vi "CalDiaVelAll.vi"() -> ()   [LabVIEW 2017]
uses:
  <vilib>/Utility/file.llb/Write Delimited Spreadsheet (string).vi
  <vilib>/Utility/file.llb/Write Delimited Spreadsheet (DBL).vi
panel:
  in  "Velocity Results File":path
  in  "Diameter Results File":path
  in  "Calibration (1 pixel = ?um)":dbl=1.45
  out "Measurment Progress":u8(slide) scale=0.0..36.0
  out "Quantifying":dbl
  out "Total Video Segments to Quantify":dbl
  # "This VI performs diameter and velocity measurements of all videos in the selected folder. The user is prompted to select the folder after which they choose a point on the top vessel wall for all the segments then a point on the bottom vessel wall. The VI then runs through all the segments and outputs the values into two text files 'Diameter' and 'Velocity'. Due to dependencies this VI is currently set to use frame 5000 as a template"
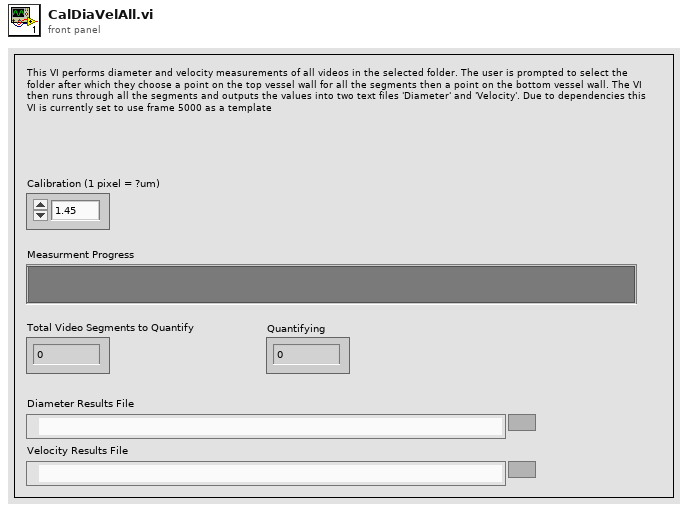
[diagram p1: front panel]
types:
  T1 = typedef "IMAQ AVI2 Refnum.ctl" = refnum<k20>
  T2 = typedef "IMAQ Image.ctl" = refnum<image>
  T3 = typedef "IMAQ Point" = cluster{"X":sgl, "Y":sgl}
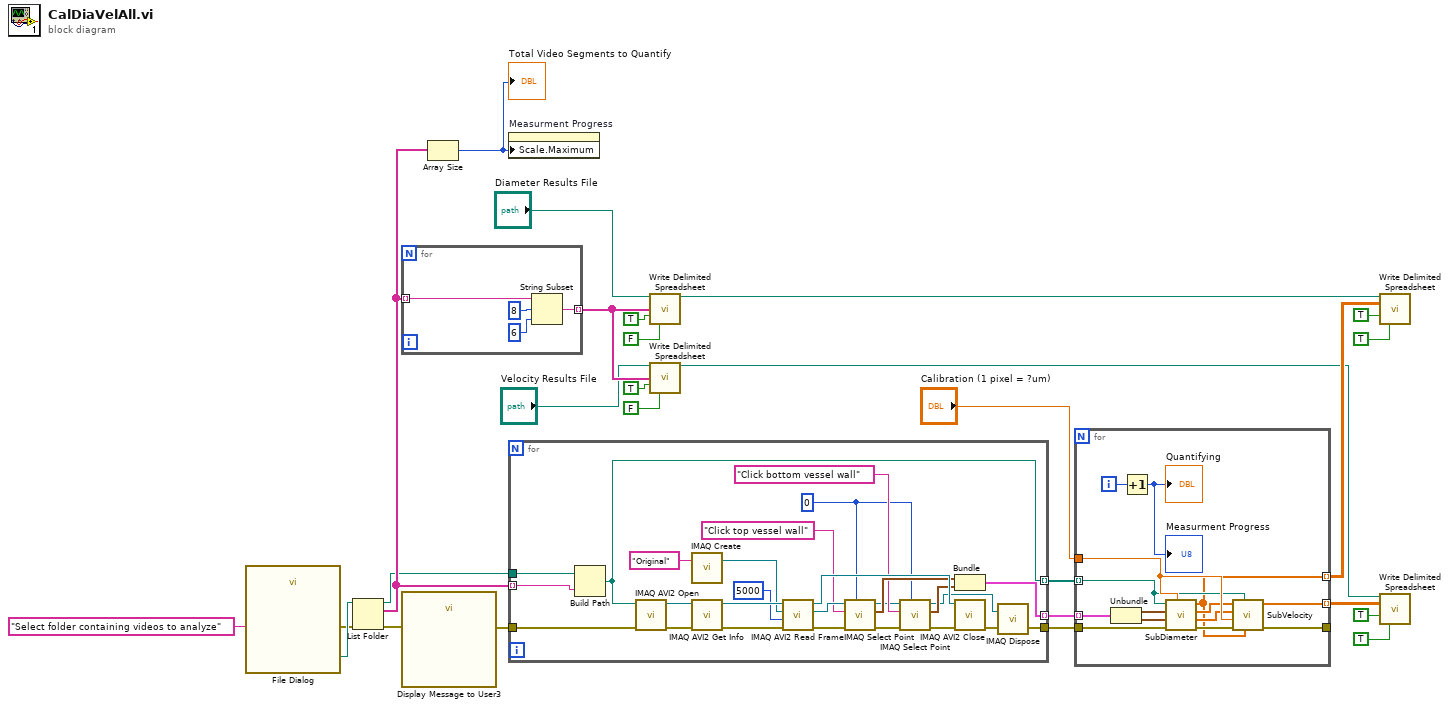
[diagram p0: block diagram]
diagram:
  n1 = call "File Dialog"("prompt"="Select folder containing videos to analyze") -> ("selected path"=w26:path, "error out"=w25:errorcluster)  [unwired: 11 in, 2 out]
  n2 = List Folder(path=w26, error in=w25) -> (path out=w9:path, filenames=w10:string[], error out=w12:errorcluster)  [unwired: 2 in, 1 out]
  n3 = for {
    tunnel: w10 -> [w31] mode=indexing
    tunnel: [w28] -> w3 mode=indexing
    n4 = String Subset(string=w31, offset (0)=8, length (rest)=6 ("length (rest)")) -> (substring=w28:string)
  }
  n5 = call "Display Message to User3"("error in (no error)"=w12) -> ("error out"=w11:errorcluster)  [unwired: 9 in, 1 out]
  n6 = Array Size(array=w10) -> (size(s)=w24:i32)
  "Total Video Segments to Quantify" <- w24
  n7 = property on="Measurment Progress" class="Slide (strict)"("Scale.Maximum"=w24) -> ()  [unwired: 2 in, 2 out]
  n8 = for {
    tunnel: [w47] -> w14
    tunnel: [w49] -> w13 mode=indexing
    tunnel: [w39] -> w15 mode=indexing
    tunnel: w11 -> [w34]
    tunnel: w10 -> [w33] mode=indexing
    tunnel: w9 -> [w32]
    w35 = 0 ("Window Number (0...15)")
    n9 = Build Path(base path=w32, name or relative path=w33) -> (appended path=w49:path)
    n10 = call "IMAQ AVI2 Open"("error in (no error)"=w34, "AVI File Path"=w49) -> ("error out"=w56:errorcluster, "AVI Refnum"=w57:T1)  [unwired: 8 in]
    n11 = call "IMAQ Create"("Image Name"="Original") -> ("New Image"=w53:T2)  [unwired: 4 in, 1 out]
    n12 = call "IMAQ AVI2 Get Info"("error in (no error)"=w56, "AVI Refnum"=w57) -> ("error out"=w52:errorcluster, "AVI Refnum (duplicate)"=w55:T1)  [unwired: 5 in, 3 out]
    n13 = call "IMAQ AVI2 Read Frame"("error in (no error)"=w52, "Frame Number"=u32 5000, "Image"=w53, "AVI Refnum"=w55) -> ("error out"=w46:errorcluster, "Image Out"=w45:T2, "AVI Refnum (duplicate)"=w50:T1)  [unwired: 5 in]
    n14 = call "IMAQ Select Point"("Window Number (0...15)"=w35, "error in (no error)"=w46, "Prompt"="Click top vessel wall", "Image In"=w45) -> ("error out"=w43:errorcluster, "Point"=w40:T3, "Image Out (duplicate)"=w36:T2)  [unwired: 4 in, 1 out]
    n15 = call "IMAQ Select Point"("Window Number (0...15)"=w35, "error in (no error)"=w43, "Prompt"="Click bottom vessel wall", "Image In"=w36) -> ("error out"=w42:errorcluster, "Point"=w41:T3, "Image Out (duplicate)"=w37:T2)  [unwired: 4 in, 1 out]
    n16 = Bundle("Point"=w40, "Point"=w41) -> (w39:cluster{"Point":T3, "Point":T3})  [unwired: 1 in]
    n17 = call "IMAQ AVI2 Close"("error in (no error)"=w42, "AVI Refnum"=w50) -> ("error out"=w48:errorcluster)  [unwired: 9 in]
    n18 = call "IMAQ Dispose"("Image"=w37, "error in (no error)"=w48) -> ("error out"=w47:errorcluster)  [unwired: 4 in]
  }
  n19 = call-poly <vilib>:"Write Delimited Spreadsheet.vi"("file path (dialog if empty)"="Diameter Results File", "1D data"=w3, "append to file? (new file:F)"=TRUE, "transpose? (no:F)"=FALSE) -> ("new file path (Not A Path if cancelled)"=w17:path)  [unwired: 10 in, 1 out]
  n20 = call-poly <vilib>:"Write Delimited Spreadsheet.vi"("file path (dialog if empty)"="Velocity Results File", "1D data"=w3, "append to file? (new file:F)"=TRUE, "transpose? (no:F)"=FALSE) -> ("new file path (Not A Path if cancelled)"=w5:path)  [unwired: 10 in, 1 out]
  n21 = for {
    tunnel: w14 -> [w71]
    tunnel: "Calibration (1 pixel = ?um)" -> [w68]
    tunnel: w15 -> [w64] mode=indexing
    tunnel: w13 -> [w61] mode=indexing
    tunnel: [w60] -> _
    tunnel: [w59] -> w4 mode=indexing
    tunnel: [w58] -> w8 mode=indexing
    i -> [w70]
    n22 = Unbundle(w64) -> ("Point"=w63:T3, "Point"=w62:T3)
    n23 = Increment(x=w70) -> (x+1=→"Quantifying" →"Measurment Progress":i32)
    n24 = call "SubDiameter.vi"("Calibration (1 pixel = ?um)"=w68, "error in (no error)"=w71, "Bot Wall"=w62, "Top wall"=w63, "AVI Path"=w61) -> ("error out"=w65:errorcluster, "Y Mid"=w66:sgl[], "X Mid"=w67:sgl[], "Diameter"=w58:dbl[])  [unwired: 3 in]
    n25 = call "SubVelocity.vi"("Vessel Diameter"=w58, "AVI Path"=w61, "error in (no error)"=w65, "Calibration factor (1 pix = ? um)"=w68, "Y"=w66, "X"=w67) -> ("error out"=w60:errorcluster, "Velocity"=w59:dbl[])  [unwired: 2 in]
  }
  n26 = call-poly <vilib>:"Write Delimited Spreadsheet.vi"("file path (dialog if empty)"=w17, "2D data"=w8, "append to file? (new file:F)"=TRUE, "transpose? (no:F)"=TRUE) -> ()  [unwired: 10 in, 2 out]
  n27 = call-poly <vilib>:"Write Delimited Spreadsheet.vi"("file path (dialog if empty)"=w5, "2D data"=w4, "append to file? (new file:F)"=TRUE, "transpose? (no:F)"=TRUE) -> ()  [unwired: 10 in, 2 out]
